vi "JoystickConditioner(SubVI).vi"(5 "DeadBand":dbl=0.15 format="%#_13g", 7 "Sensitivity":dbl=1.0 format="%#_13g", 9 "joystick axis":dbl format="%#_13g") -> (1 "output":dbl)   [LabVIEW 2019, in "Joysticks.lvlib" / "Joysticks.lvclass"]
doc: "Applies deadband and scales it to the joystick."
uses:
  Joysticks.lvclass
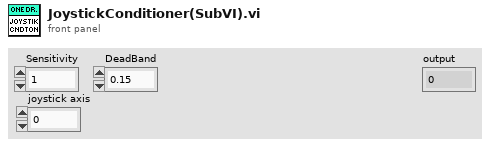
[diagram p1: front panel]
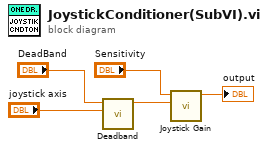
[diagram p0: block diagram]
diagram:
  n1 = call "Deadband.vi"("joystick axis"="joystick axis", "DeadBand"="DeadBand") -> ("Deadbanded output"=w5:dbl)  [unwired: 9 in]
  n2 = call "Joystick Gain.vi"("input"=w5, "Sensitivity"="Sensitivity") -> ("output"=→"output":dbl)  [unwired: 9 in]
